vi "Trig OP Setup-unpack.vi"(8 "Values":dbl[](array[numeric]), 9 "Keys setup":T3=[{"key"="Control FPGA.MAC address", "Save?"=TRUE, "Default"="AABBCCDDEEFF"}, {"key"="DAQ FPGA.Target", "Save?"=TRUE, "Default"="RIO0"}, {"key"="XY Stage.COM port", "Save?"=TRUE, "Default"="COM7"}, {"key"="DAQmx Chan.Pockels Control", "Save?"=TRUE, "Default"=""}, {"key"="DAQmx Chan.Hard Shutter", "Save?"=TRUE, "Default"=""}, {"key"="DAQmx Chan.PMT 1", "Save?"=TRUE, "Default"=""}, {"key"="DAQmx Chan.PMT 2", "Save?"=TRUE, "Default"=""}, {"key"="DAQmx Chan.Encoder Trigger", "Save?"=TRUE, "Default"=""}, {"key"="DAQmx Chan.Optional Trigger 1", "Save?"=TRUE, "Default"=""}, {"key"="DAQmx Chan.Optional Trigger 2", "Save?"=TRUE, "Default"=""}, {"key"="DAQmx Chan.Optional Trigger 3", "Save?"=TRUE, "Default"=""}], 11 "Value read/used":string[](array[string])) -> (0 "output cluster":T1={"Trigger 1 function"=enum."Encoder trigger", "Triggers loop clock (MHz)"=80.0} {"Triggers loop clock (MHz)" format="%#_13g"}, 3 "Triggers output setup":T4 {"Pulse width (us)" min=10 max=5000 step=1 format="%.0fµs"})   [LabVIEW 2017]
uses:
  Peripherals Control/Triggers/Typedefs/Triggers output setup.ctl
  Peripherals Control/Triggers/Typedefs/Trigger setup element cluster.ctl
  Typedefs/Ini file interface (String).ctl
  Peripherals Control/Triggers/Typedefs/General trigger settings cluster.ctl
  Typedefs/Trigger 1 selector enum.ctl
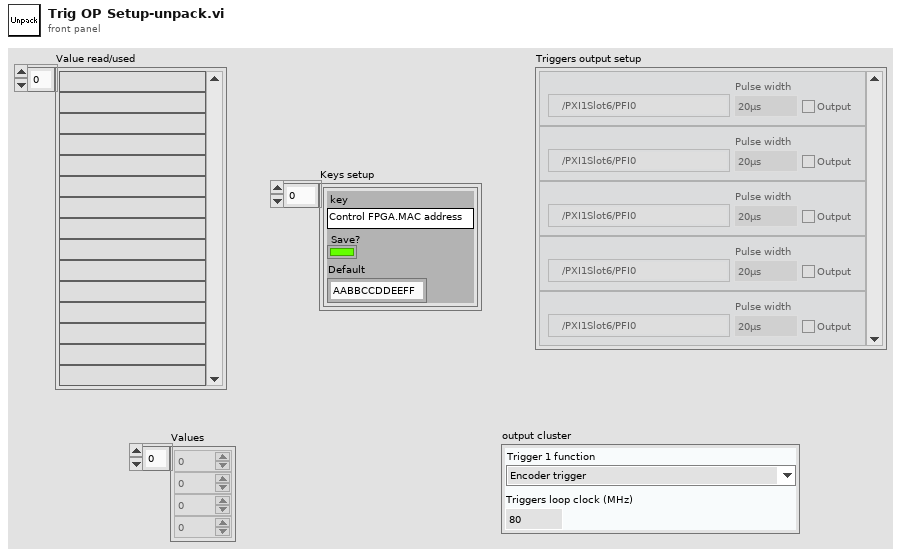
[diagram p1: front panel]
types:
  T1 = typedef "General trigger settings cluster.ctl" = cluster{"Trigger 1 function":T2, "Triggers loop clock (MHz)":dbl}
  T2 = typedef "Trigger 1 selector enum.ctl" = enum16{"Encoder trigger", "Line trigger", "Control system's ref frame acknowledgement"}
  T3 = typedef "Ini file interface (String).ctl" = cluster{"key":string, "Save?":bool, "Default":string}[]
  T4 = typedef "Triggers output setup.ctl" = T5[]
  T5 = typedef "Trigger setup element cluster.ctl" = cluster{"Name":string, "Output?":bool, "Output terminal":tag, "PXI backplane line":tag, "Pulse width (us)":u16}
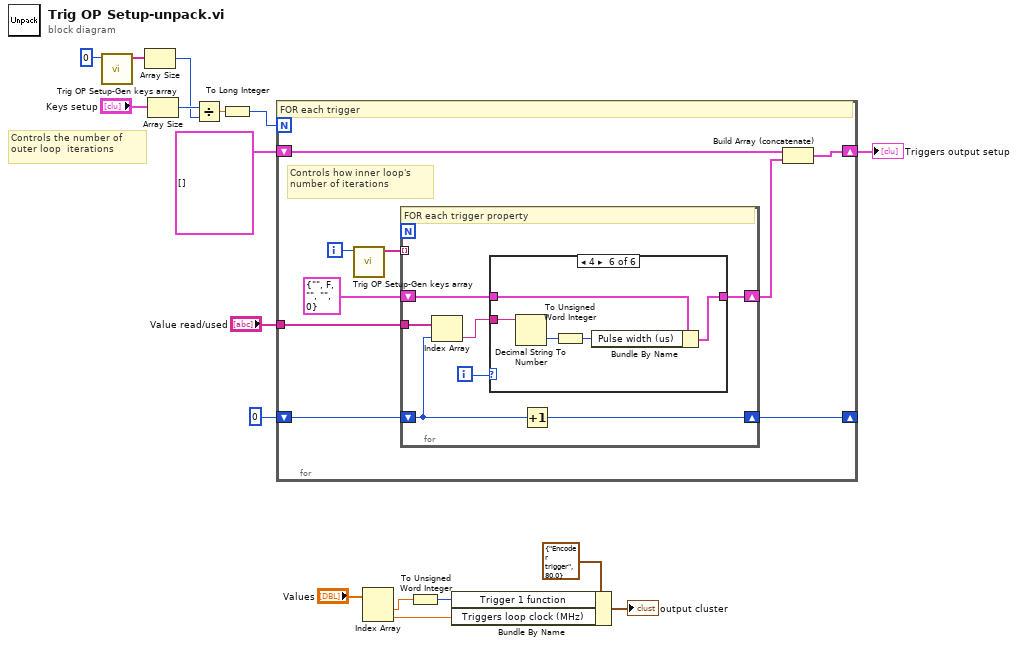
[diagram p0: block diagram]
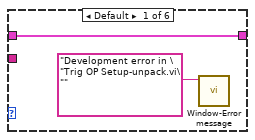
[diagram p2: hidden frame]
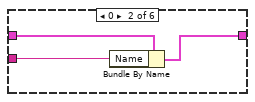
[diagram p3: hidden frame]
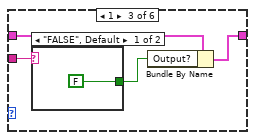
[diagram p4: hidden frame]
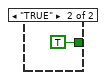
[diagram p5: hidden frame]
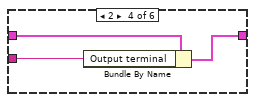
[diagram p6: hidden frame]
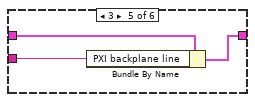
[diagram p7: hidden frame]
diagram:
  # "Controls the number of outer loop  iterations"
  n1 = call "Trig OP Setup-Gen keys array.vi"("Trigger index (FOR loop index)"=0) -> ("Keys array for each trigger"=w12:string[])  [unwired: 10 in]
  n2 = Array Size(array=w12) -> (size(s)=w9:i32)
  n3 = Array Size(array="Keys setup") -> (size(s)=w10:i32)
  n4 = Divide(x=w10, y=w9) -> (x/y=w8:dbl)
  n5 = To Long Integer(number=w8) -> (32bit integer=w7:i32)
  n6 = for {
    N: w7 -> [_]
    tunnel: "Value read/used" -> [w20]
    shift-right: [w23] -> w15
    shift-left: T4 [] ("Triggers output setup") -> [w24]
    shift-right: [w19] -> _
    shift-left: 0 -> [w18]
    i -> [w26]
    # "Controls how inner loop's number of iterations"
    # "FOR each trigger"
    n7 = call "Trig OP Setup-Gen keys array.vi"("Trigger index (FOR loop index)"=w26) -> ("Keys array for each trigger"=w25:string[])  [unwired: 10 in]
    n8 = for {
      tunnel: w25 -> [_] mode=indexing
      shift-right: [w33] -> w22
      shift-left: T5 {"Name"="", "Output?"=FALSE, "Output terminal"="", "PXI backplane line"="", "Pulse width (us)"=0} ("Trigger setup element") -> [w32]
      tunnel: w20 -> [w30]
      shift-right: [w29] -> w19
      shift-left: w18 -> [w28]
      i -> [w31]
      # "FOR each trigger property"
      n9 = Index Array(array=w30, index=w28) -> (element=w27:string)
      n10 = case shown="4" w31 {
        tunnel: [w35 w38 w41 w46 w49 w54] -> w33
        tunnel: w32 -> [w35 w37 w42 w47 w50 w55]
        tunnel: w27 -> [_ w36 w40 w45 w48 w53]
        frame Default {
          n11 = call "Window-Error message.vi"("Message"="Development error in \"Trig OP Setup-unpack.vi\"" ("Error Message")) -> ()  [unwired: 10 in, 1 out]
        }
        frame 0 {
          n12 = Bundle By Name(cluster=w37, "Name"=w36) -> (w38:T5)
        }
        frame 1 {
          n13 = case shown="\"FALSE\", Default" w40 {
            tunnel: [FALSE TRUE] -> w39
            frame "FALSE", Default {
            }
            frame "TRUE" {
            }
          }
          n14 = Bundle By Name(cluster=w42, "Output?"=w39) -> (w41:T5)
        }
        frame 2 {
          n15 = Bundle By Name(cluster=w47, "Output terminal"=w45) -> (w46:T5)
        }
        frame 3 {
          n16 = Bundle By Name(cluster=w50, "PXI backplane line"=w48) -> (w49:T5)
        }
        frame 4 {
          n17 = Decimal String To Number(string=w53) -> (number=w52:i32)  [unwired: 2 in, 1 out]
          n18 = To Unsigned Word Integer(number=w52) -> (unsigned 16bit integer=w51:u16)
          n19 = Bundle By Name(cluster=w55, "Pulse width (us)"=w51) -> (w54:T5)
        }
      }
      n20 = Increment(x=w28) -> (x+1=w29:i32)
    }
    n21 = Build Array (concatenate)(w24, w22) -> (w23:T4)
  }
  "Triggers output setup" <- w15
  n22 = Index Array(array="Values") -> (element #1=w5:dbl, element #2=w4:dbl)  [unwired: 2 in]
  n23 = To Unsigned Word Integer(number=w5) -> (unsigned 16bit integer=w1:u16)
  n24 = Bundle By Name(cluster=T1 {"Trigger 1 function"=enum."Encoder trigger", "Triggers loop clock (MHz)"=80.0} ("General trigger settings"), "Trigger 1 function"=w1, "Triggers loop clock (MHz)"=w4) -> (→"output cluster":T1)
